vi "Insert Value (Value[]).vi"(7 "keys":string[](array[string]), 8 "error in (no error)":errorcluster, 10 "values":refnum<class "JSON Value.lvclass">[](array[class]), 11 "JSON Value in":refnum<class "JSON Value.lvclass">) -> (0 "error out":errorcluster, 1 "replaced?":bool[](array[boolean]), 3 "JSON Value out":refnum<class "JSON Value.lvclass">)   [LabVIEW 2016, in "JSON Value.lvclass"]
uses:
  JSON Value.lvclass
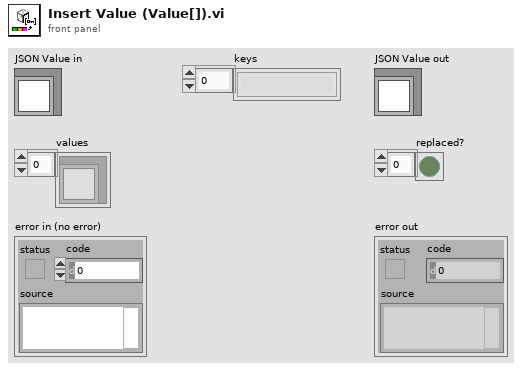
[diagram p1: front panel]
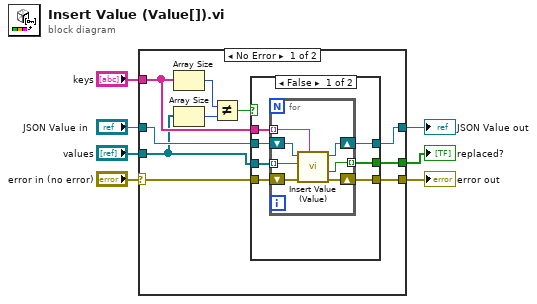
[diagram p0: block diagram]
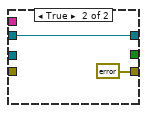
[diagram p2: hidden frame]
diagram:
  n1 = case shown="No Error" "error in (no error)" {
    selector: "error in (no error)" -> [w14 w35]
    tunnel: [w13 w35] -> w6
    tunnel: [w11 w34] -> w4
    tunnel: "JSON Value in" -> [w12 w34]
    tunnel: "keys" -> [w10 _]
    tunnel: "values" -> [w9 _]
    tunnel: [w8 _] -> w1
    frame No Error {
      n2 = Array Size(array=w10) -> (size(s)=w17:i32)
      n3 = Array Size(array=w9) -> (size(s)=w16:i32)
      n4 = Not Equal?(x=w17, y=w16) -> (x != y?=w15:bool)
      n5 = case shown="False" w15 {
        tunnel: w14 -> [w22 _]
        tunnel: [w21 errorcluster {"status"=TRUE, "code"=-1000, "source"="There must be an equal number of keys and values"} ("error constant")] -> w13
        tunnel: w12 -> [w24 w32]
        tunnel: [w23 w32] -> w11
        tunnel: w10 -> [w20 _]
        tunnel: w9 -> [w19 _]
        tunnel: [w18 _] -> w8
        frame False {
          n6 = for {
            shift-right: [w30] -> w23
            shift-left: w24 -> [w31]
            shift-right: [w28] -> w21
            shift-left: w22 -> [w29]
            tunnel: w20 -> [w27] mode=indexing
            tunnel: w19 -> [w26] mode=indexing
            tunnel: [w25] -> w18 mode=indexing
            n7 = call "Insert Value (Value).vi"("key"=w27, "error in (no error)"=w29, 10:"JSON Value in"=w26, 11:"JSON Value in"=w31) -> ("error out"=w28:errorcluster, "replaced"=w25:bool, "JSON Value out"=w30:refnum<class "JSON Value.lvclass">)  [unwired: 5 in]
          }
        }
        frame True {
        }
      }
    }
    frame Error {
    }
  }
  "error out" <- w6
  "JSON Value out" <- w4
  "replaced?" <- w1
